vi "FormatTester.vi"() -> ()   [LabVIEW 2015]
panel:
  out "spreadsheet string":string
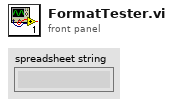
[diagram p1: front panel]
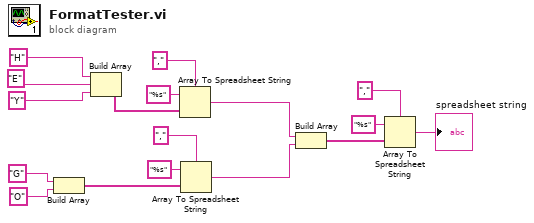
[diagram p0: block diagram]
diagram:
  n1 = Build Array("G", "O") -> (w7:string[])
  n2 = Build Array("H", "E", "Y") -> (w14:string[])
  n3 = Array To Spreadsheet String(delimiter (Tab)=",", array=w14, 3:"%s" ("format string")) -> (spreadsheet string=w3:string)
  n4 = Array To Spreadsheet String(delimiter (Tab)=",", array=w7, 3:"%s" ("format string")) -> (spreadsheet string=w2:string)
  n5 = Build Array(w3, w2) -> (w4:string[])
  n6 = Array To Spreadsheet String(delimiter (Tab)=",", array=w4, 3:"%s" ("format string")) -> (spreadsheet string=→"spreadsheet string":string)
